vi "FP_Control Property Set from Ref Array.vi"(7 "Panel":refnum<vi>, 8 "Error":errorcluster, 9 "FP Ctrl Properies":T1, 11 "FP Controls":refnum<vi>[](array[refnum])) -> (0 "Error Out":errorcluster, 3 "Success Out":bool)   [LabVIEW 2015]
uses:
  TypeDefs_Utility/ENUM_FP_Hide Show Disable.ctl
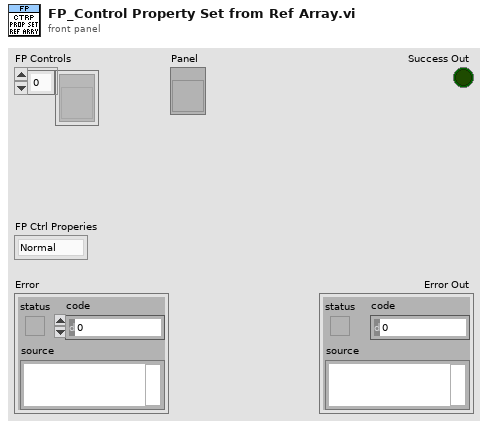
[diagram p1: front panel]
types:
  T1 = typedef "ENUM_FP_Hide Show Disable.ctl" = enum16{"Normal", "Disable", "Disable Gray", "Hide"}
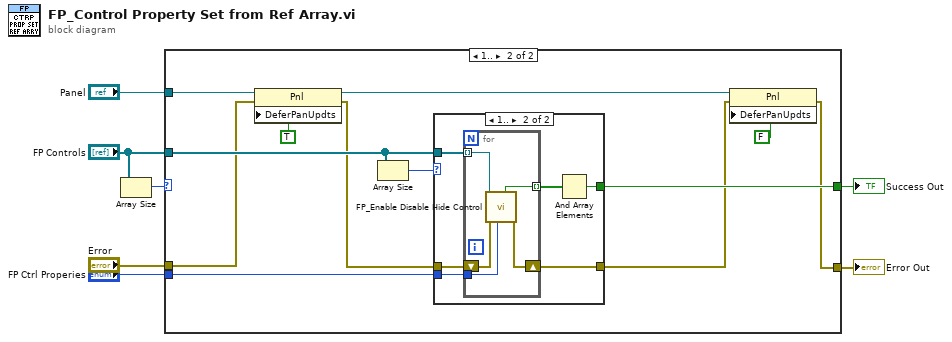
[diagram p0: block diagram]
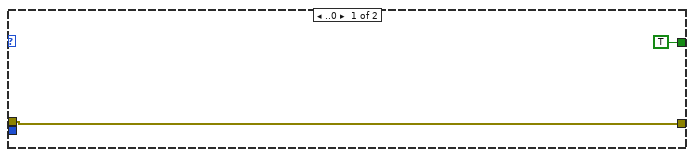
[diagram p2: hidden frame]
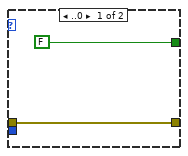
[diagram p3: hidden frame]
diagram:
  n1 = Array Size(array="FP Controls") -> (size(s)=w1:i32)
  n2 = case shown="1.." w1 {
    tunnel: [TRUE w21] -> w7
    tunnel: "FP Controls" -> [_ w19]
    tunnel: "Error" -> [w8 w18]
    tunnel: "Panel" -> [_ w17]
    tunnel: "FP Ctrl Properies" -> [_ w14]
    tunnel: [w8 w12] -> w3
    frame ..0 {
    }
    frame 1.. {
      n3 = property class="Pnl"(reference=w17, error in=w18, "DeferPanUpdts"=TRUE ("Defer Panel Updates")) -> (reference out=w11:refnum<vi>, error out=w15:errorcluster)
      n4 = Array Size(array=w19) -> (size(s)=w20:i32)
      n5 = case shown="1.." w20 {
        tunnel: w14 -> [_ w29]
        tunnel: w15 -> [w23 w28]
        tunnel: [w23 w27] -> w16
        tunnel: [FALSE w24] -> w21
        tunnel: w19 -> [_ w26]
        frame ..0 {
        }
        frame 1.. {
          n6 = for {
            tunnel: w29 -> [w34]
            tunnel: w26 -> [w30] mode=indexing
            tunnel: [w31] -> w25 mode=indexing
            shift-right: [w33] -> w27
            shift-left: w28 -> [w32]
            n7 = call "FP_Enable Disable Hide Control.vi"("Settings"=w34, "Error"=w32, "Ctl Refnum"=w30) -> ("Error Out"=w33:errorcluster, "Success"=w31:bool)  [unwired: 4 in, 3 out]
          }
          n8 = And Array Elements(Boolean array=w25) -> (logical AND=w24:bool)
        }
      }
      n9 = property class="Pnl"(reference=w11, error in=w16, "DeferPanUpdts"=FALSE ("Defer Panel Updates")) -> (error out=w12:errorcluster)  [unwired: 1 out]
    }
  }
  "Success Out" <- w7
  "Error Out" <- w3
